vi "Read_Array.vi"(8 "error in (no error)":errorcluster, 9 "Range 2 to Read":string="C2", 10 "Range 1 to Read":string="C2", 11 "Automation Refnum in":refnum<k7>) -> (0 "error out":errorcluster, 2 "Read Values Array":dbl[][](array[numeric]), 3 "reference out":refnum<k7>)   [LabVIEW 2014]
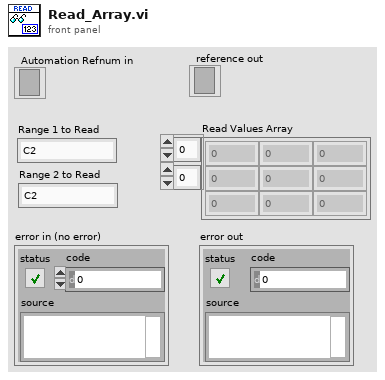
[diagram p1: front panel]
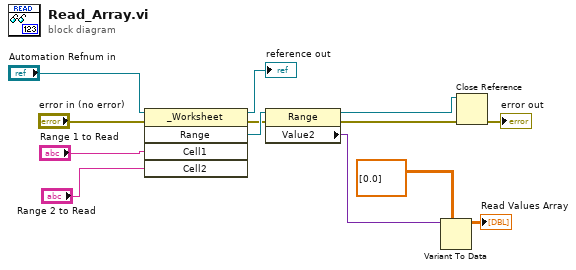
[diagram p0: block diagram]
diagram:
  n1 = invoke class="_Worksheet" method="Range"(reference="Automation Refnum in", error in="error in (no error)", "Cell1"="Range 1 to Read", "Cell2"="Range 2 to Read") -> (reference out=→"reference out":refnum<k7>, error out=w8:errorcluster, "Range"=w9:refnum<k7>)  [unwired: 1 in, 2 out]
  n2 = property class="Range"(reference=w9, error in=w8) -> (reference out=w6:refnum<k7>, error out=w5:errorcluster, "Value2"=w10:variant)
  n3 = Variant To Data(type=dbl[][] [[0.0]], Variant=w10) -> (data=→"Read Values Array":dbl[][])  [unwired: 1 in, 1 out]
  n4 = Close Reference(reference=w6, error in (no error)=w5) -> (error out=→"error out":errorcluster)
